vi "Micron Optics sm130 Triggered Acquisition.vi"() -> ()   [LabVIEW 2024]
doc: "Demonstrates the triggered peak wavelength acquisition. The peak wavelength acquisition can be untriggered, software or hardware triggered. \n\n<b>Note:</b>\nThis example is made for the instrument without channel multiplexer. Modifications will have to be made for instruments with channel multiplexer."
uses:
  Micron Optics sm130.lvlib
panel:
  in  "Trigger Type (0:Untriggered)":u16(ring) items=["Untriggered", "Software Triggered", "Hardware Triggered"]
  in  "Sensor Number (1)":i32=1
  in  "Channel (1: Channel 1)":i32(ring)=1 items=["Channel 1"=1, "Channel 2"=2, "Channel 3"=3, "Channel 4"=4]
  out "Peak Wavelength Chart":dbl(graph)
  in  "Stop":bool
  in  "Stop Trigger":bool
  in  "Start Trigger":bool
  in  "Data Interleave (1)":i32=1
  in  "Number of Acquisitions (100)":i32=100
  in  "Trigger Stop Condition (1:Edge Triggering)":u16(ring)=1 items=["Number of Acquisitions", "Edge Triggering"]
  in  "Trigger Stop Edge (0: Rising)":u16(ring) items=["Rising", "Falling"]
  in  "Trigger Start Edge (0: Rising)":u16(ring) items=["Rising", "Falling"]
  in  "VISA resource name":refnum<visa-resource-name>
  # "(c) 2009 - 2012 National Instruments.  ALL RIGHTS RESERVED."
  # "Sensor View"
  # "Trigger Control"
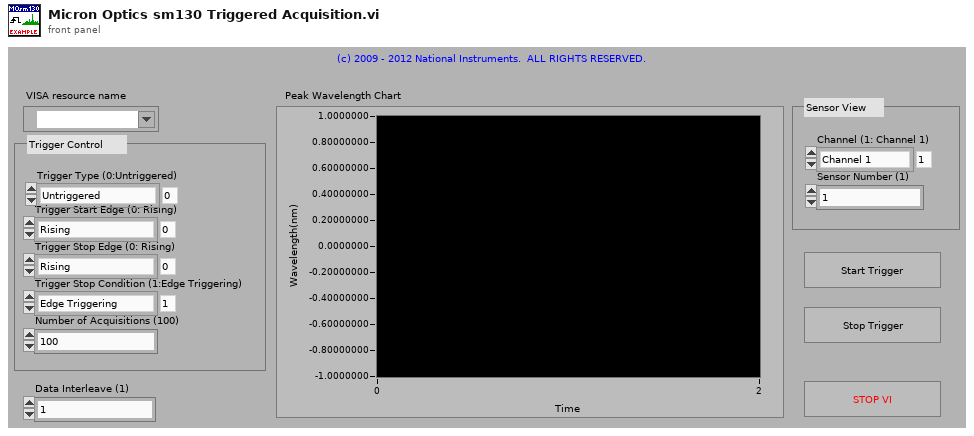
[diagram p1: front panel]
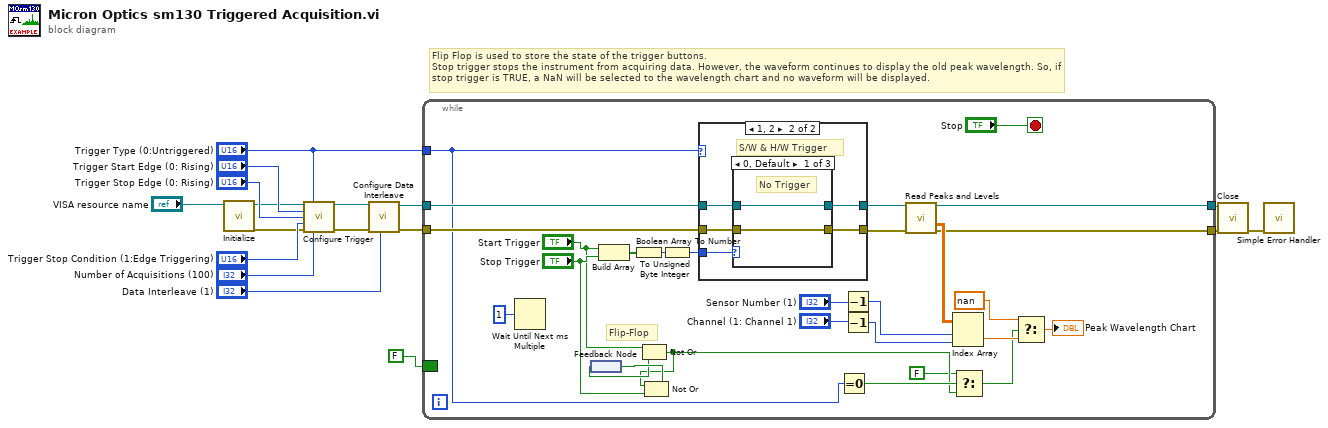
[diagram p0: block diagram]
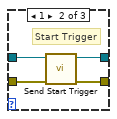
[diagram p3: hidden frame]
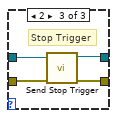
[diagram p4: hidden frame]
diagram:
  # "Flip Flop is used to store the state of the trigger buttons. \nStop trigger stops the instrument from acquiring data. However, the waveform continues to display the old peak wavelength. So, if stop trigger is TRUE, a NaN will be selected to the wavelength chart and no waveform will be displayed."
  n1 = call "Initialize.vi"("VISA resource name"="VISA resource name") -> ("error out"=w8:errorcluster, "VISA resource name out"=w9:refnum<visa-resource-name>)  [unwired: 9 in]
  n2 = call "Configure Trigger.vi"("VISA resource name"=w9, "Trigger Type (0:Untriggered)"="Trigger Type (0:Untriggered)", "Trigger Start Edge (0: Rising)"="Trigger Start Edge (0: Rising)", "Trigger Stop Edge (0: Rising)"="Trigger Stop Edge (0: Rising)", "Trigger Stop Condition (1:Edge Triggering)"="Trigger Stop Condition (1:Edge Triggering)", "error in (no error)"=w8, "Number of Acquisitions (100)"="Number of Acquisitions (100)") -> ("VISA resource name out"=w12:refnum<visa-resource-name>, "error out"=w11:errorcluster)  [unwired: 6 in, 1 out]
  n3 = call "Configure Data Interleave.vi"("Data Interleave (1)"="Data Interleave (1)", "error in (no error)"=w11, "VISA resource name"=w12) -> ("error out"=w5:errorcluster, "VISA resource name out"=w6:refnum<visa-resource-name>)  [unwired: 7 in]
  n4 = while {
    tunnel: w6 -> [w40]
    tunnel: w5 -> [w42]
    tunnel: "Trigger Type (0:Untriggered)" -> [w20]
    tunnel: [w25] -> w4
    tunnel: [w24] -> w3
    border: FALSE -> [_]
    stop <- "Stop" stop-if-true
    # "Flip-Flop"
    n5 = Wait Until Next ms Multiple(millisecond multiple=u32 1) -> ()  [unwired: 1 out]
    n6 = feedback #1() -> (w28:bool)
    n7 = Build Array("Start Trigger", "Stop Trigger") -> (w45:bool[])
    n8 = Boolean Array To Number(Boolean array=w45) -> (number=w44:u32)
    n9 = Not Or(1:w28, 2:"Start Trigger") -> (0:w21:bool)
    n10 = Not Or(1:"Stop Trigger", 2:w21) -> (0:w29:bool)
    n11 = feedback-in #1(w29) -> ()
    n12 = To Unsigned Byte Integer(number=w44) -> (unsigned 8bit integer=w43:u8)
    n13 = case shown="1, 2" w20 {
      tunnel: w43 -> [_ w52]
      tunnel: w40 -> [w47 w51]
      tunnel: w42 -> [w46 w50]
      tunnel: [w46 w49] -> w37
      tunnel: [w47 w48] -> w38
      frame 0, Default {
        # "Untriggered"
      }
      frame 1, 2 {
        # "S/W & H/W Trigger"
        n14 = case shown="0, Default" w52 {
          tunnel: w51 -> [w54 w58 w62]
          tunnel: w50 -> [w53 w57 w59]
          tunnel: [w54 w56 w61] -> w48
          tunnel: [w53 w55 w60] -> w49
          frame 0, Default {
            # "No Trigger"
          }
          frame 1 {
            # "Start Trigger"
            n15 = call "Send Start Trigger.vi"("error in (no error)"=w57, "VISA resource name"=w58) -> ("error out"=w55:errorcluster, "VISA resource name out"=w56:refnum<visa-resource-name>)  [unwired: 8 in]
          }
          frame 2 {
            # "Stop Trigger"
            n16 = call "Send Stop Trigger.vi"("error in (no error)"=w59, "VISA resource name"=w62) -> ("error out"=w60:errorcluster, "VISA resource name out"=w61:refnum<visa-resource-name>)  [unwired: 8 in]
          }
        }
      }
    }
    n17 = Equal To 0?(x=w20) -> (x = 0?=w22:bool)
    n18 = Decrement(x="Sensor Number (1)") -> (x-1=w33:i32)
    n19 = Decrement(x="Channel (1: Channel 1)") -> (x-1=w32:i32)
    n20 = call "Read Peaks and Levels.vi"("VISA resource name"=w38, "error in (no error)"=w37) -> ("VISA resource name out"=w25:refnum<visa-resource-name>, "Peak Wavelengths (nm)"=w36:dbl[][], "error out"=w24:errorcluster)  [unwired: 5 in, 6 out]
    n21 = Index Array(array=w36, index (row)=w33, index (col)=w32) -> (element=w30:dbl)
    n22 = Select(t=FALSE, s=w22, f=w21) -> (s? t:f=w23:bool)
    n23 = Select(t=nan, s=w23, f=w30) -> (s? t:f=→"Peak Wavelength Chart":dbl)
  }
  n24 = call "Close.vi"("error in (no error)"=w3, "VISA resource name"=w4) -> ("error out"=w2:errorcluster)  [unwired: 9 in]
  n25 = call <vilib>:"Simple Error Handler.vi"("error in (no error)"=w2) -> ()  [unwired: 4 in, 5 out]
